vi "LWXPS_GroupMotorMatrixTrace.vi"(6 "LabVIEW error IN":errorcluster, 7 "Title Trace":string, 8 "Group Name":string, 9 "XPS Reference IN":refnum<k24>) -> (0 "LabVIEW error OUT":errorcluster, 1 "XPS Error String":string, 2 "Returned error code":i32, 3 "XPS Reference OUT":refnum<k24>)   [LabVIEW 2014]
uses:
  D:/XPSQ8_LabView_Library/Development/Source/Dll/Newport.XPS.CommandInterface.dll
  Dll/Newport.XPS.CommandInterface.dll
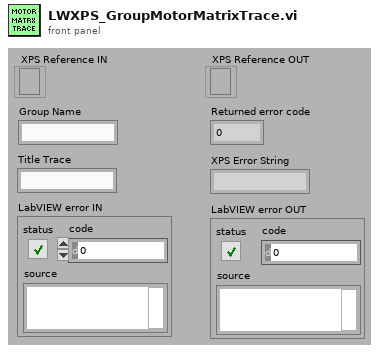
[diagram p1: front panel]
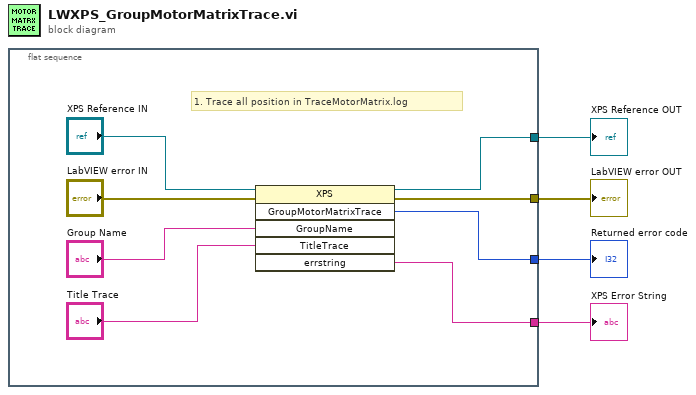
[diagram p0: block diagram]
diagram:
  n1 = flat-sequence {
    tunnel: [w10] -> w4
    tunnel: [w8] -> w3
    tunnel: [w11] -> w2
    tunnel: [w6] -> w1
    frame #0 {
      # "1. Trace all position in TraceMotorMatrix.log"
      n2 = invoke class="XPS" method="GroupMotorMatrixTrace"(reference="XPS Reference IN", error in="LabVIEW error IN", "GroupName"="Group Name", "TitleTrace"="Title Trace") -> (reference out=w10:refnum<k24>, error out=w8:errorcluster, "GroupMotorMatrixTrace"=w11:i32, "errstring"=w6:string)  [unwired: 2 in, 2 out]
    }
  }
  "XPS Reference OUT" <- w4
  "LabVIEW error OUT" <- w3
  "Returned error code" <- w2
  "XPS Error String" <- w1
